vi "Lights.vi"() -> ()   [LabVIEW 2016]
doc: "ADXL362 SPI Accelerometer\n\nThis example shows how to use the Analog Devices ADXL362 Accelerometer sensor connected to SPI.\n\nThis example expects a USB cable connected from your development PC to the Type B USB Jack (next to the power input) on the roboRIO."
uses:
  <vilib>/Rock Robotics/SystemInterfaces/spilib/spi_bus.ctl
  <vilib>/Rock Robotics/WPI/SPI/WPI_SPIMode.ctl
  Robot Global Data.vi
panel:
  in  "Blink Rate":u32=100
  in  "Global Max\nBrightness":u8(slide)=16 max=31 scale=0.0..31.0
  in  "Number ON":u8=26
  in  "Chip Select Active High (F)":bool
  in  "Mode (3)":T1=enum."Mode 3 (Clk Idle High,Sample on Trailing)"
  in  "Clock Rate (Hz)":dbl=500000.0
  in  "error in":errorcluster
  in  "SPI Bus":T2=enum."SPI On-Board, CS1"
  out "error out":errorcluster
  in  "stop":bool
  # "Set these inputs before running."
  # "Number of Lights"
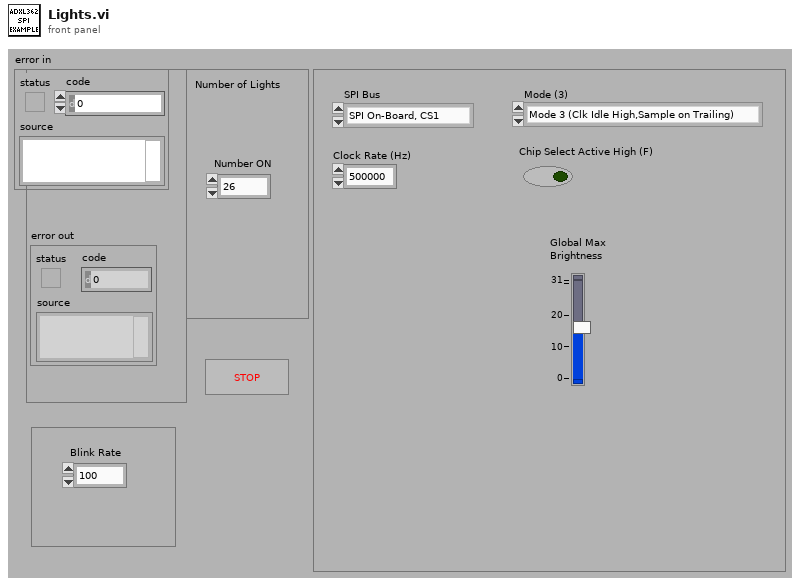
[diagram p1: front panel]
types:
  T1 = typedef "WPI_SPIMode.ctl" = enum16{"Mode 0 (Clk Idle Low,Sample on Leading)", "Mode 1 (Clk Idle Low,Sample on Trailing)", "Mode 2 (Clk Idle High,Sample on Leading)", "Mode 3 (Clk Idle High,Sample on Trailing)"}
  T2 = typedef "spi_bus.ctl" = enum16{"SPI On-Board, CS0", "SPI On-Board, CS1", "SPI On-Board, CS2", "SPI On-Board, CS3", "SPI MXP", "Invalid"}
  T3 = typedef "WPI_SPIDevRef.ctl" = cluster{"DevStatus":errorcluster, "Handle":i32, "SPI Bus":T2}
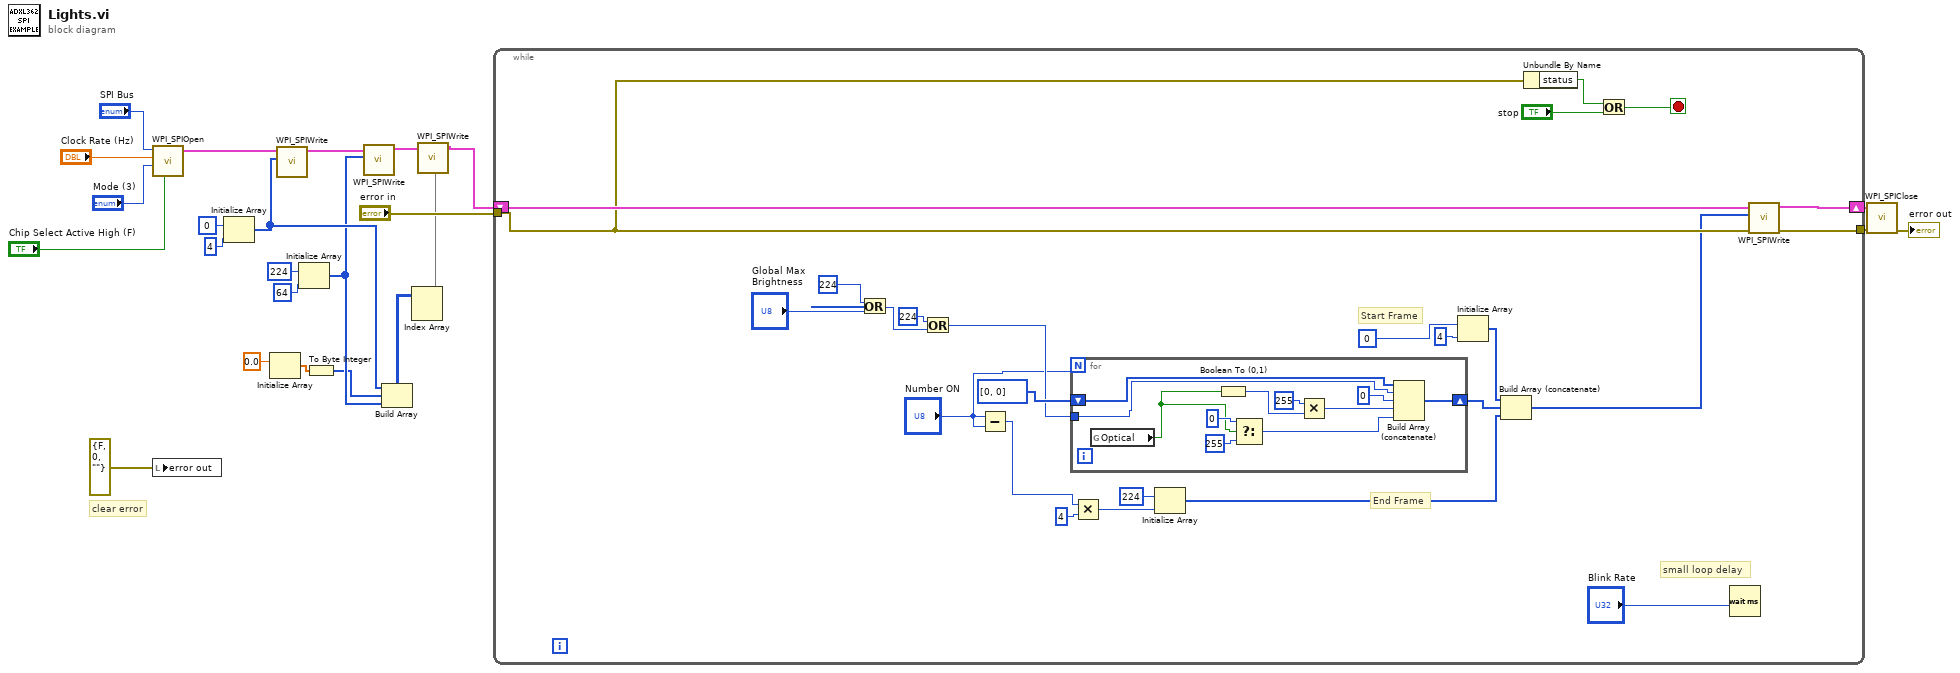
[diagram p0: block diagram]
diagram:
  # "clear error"
  n1 = call <vilib>:"WPI_SPIOpen.vi"("Chip Select Active High (F)"="Chip Select Active High (F)", "Mode (3)"="Mode (3)", "Clock Rate (Hz)"="Clock Rate (Hz)", "SPI Bus"="SPI Bus") -> ("SPIDevRef"=w14:T3)  [unwired: 6 in, 1 out]
  n2 = local write "error out"(errorcluster {"status"=FALSE, "code"=0, "source"=""} ("error out")) -> ()
  n3 = Initialize Array(u8 0 ("Data To Send"), u8 4 ("dimension size")) -> (w9:u8[])
  n4 = Initialize Array(0.0 ("element")) -> (w4:dbl[])  [unwired: 1 in]
  n5 = call <vilib>:"WPI_SPIWrite.vi"("Data To Send"=w9, "SPIDevRef"=w14) -> ("SPIDevRef"=w10:T3)  [unwired: 7 in, 2 out]
  n6 = Initialize Array(u8 224 ("Data To Send"), u8 64 ("dimension size")) -> (w8:u8[])
  n7 = To Byte Integer(number=w4) -> (8bit integer=w3:i8[])
  n8 = call <vilib>:"WPI_SPIWrite.vi"("Data To Send"=w8, "SPIDevRef"=w10) -> ("SPIDevRef"=w6:T3)  [unwired: 7 in, 2 out]
  n9 = Build Array(w9, w3, w8) -> (w2:u8[][])
  n10 = Index Array(array=w2) -> (element=w1:u8[])  [unwired: 2 in]
  n11 = call <vilib>:"WPI_SPIWrite.vi"("Data To Send"=w1, "SPIDevRef"=w6) -> ("SPIDevRef"=w7:T3)  [unwired: 7 in, 2 out]
  n12 = while {
    shift-right: [w48] -> w21
    shift-left: w7 -> [w44]
    tunnel: "error in" -> [w42]
    tunnel: [w47] -> w11
    stop <- w41 stop-if-true
    # "End Frame"
    # "Start Frame"
    # "small loop delay"
    n13 = Or(x=u8 224, y="Global Max\nBrightness") -> (x .or. y?=w25:u8)
    n14 = Or(x=u8 224, y=w25) -> (x .or. y?=w29:u8)
    n15 = Subtract(x="Number ON", y="Number ON") -> (x-y=w33:u8)
    n16 = for {
      N: "Number ON" -> [_]
      tunnel: w29 -> [w56]
      shift-right: [w52] -> w38
      shift-left: i16[] [0, 0] -> [w51]
      n17 = global read "Robot Global Data.vi" "Optical"() -> (w50:bool)
      n18 = Boolean To (0,1)(Boolean=w50) -> (0, 1=w59:i16)
      n19 = Select(t=u8 0, s=w50, f=u8 255) -> (s? t:f=w53:u8)
      n20 = Multiply(x=u8 255, y=w59) -> (x*y=w54:i16)
      n21 = Build Array (concatenate)(w51, w56, u8 0 ("element"), w54, w53) -> (w52:i16[])
    }
    n22 = Multiply(x=w33, y=4) -> (x*y=w35:i32)
    n23 = Initialize Array(u8 224 ("Data To Send"), w35) -> (w37:u8[])
    n24 = Initialize Array(u8 0 ("Data To Send"), u8 4 ("dimension size")) -> (w36:u8[])
    n25 = Build Array (concatenate)(w36, w38, w37) -> (w27:i16[])
    n26 = Unbundle By Name(w42) -> ("status"=w43:bool)
    n27 = Or(x=w43, y="stop") -> (x .or. y?=w41:bool)
    n28 = Wait (ms)(milliseconds to wait="Blink Rate") -> ()  [unwired: 1 out]
    n29 = call <vilib>:"WPI_SPIWrite.vi"("error in (no error)"=w42, "Data To Send"=w27, "SPIDevRef"=w44) -> ("error out"=w47:errorcluster, "SPIDevRef"=w48:T3)  [unwired: 6 in, 1 out]
  }
  n30 = call <vilib>:"WPI_SPIClose.vi"("error in (no error)"=w11, "SPIDevRef"=w21) -> ("error out"=→"error out":errorcluster)  [unwired: 9 in]
